vi "Skip Fire Write.vi"(0 "Device Inputs":dbl[](array[numeric]), 11 "Setup Indexes":T2[](array[typedef])) -> (6 "Setup":T1[](array[typedef]))   [LabVIEW 2016, in "DCM Engine.lvlib"]
uses:
  DCM Engine.lvlib
  Shared/Types/Skip Fire Setup Indexes.ctl
  Built/DCM Classes Packed/Pharlap/C/DCM-Classes.lvlibp/DCM/Skip Fire/RT/Skip Fire Setup.ctl
  Built/DCM Classes Packed/Pharlap/C/DCM-Classes.lvlibp/DCM/Skip Fire/RT/DCM - RT - Skip Fire.lvlib
  DCM Shared.lvlib
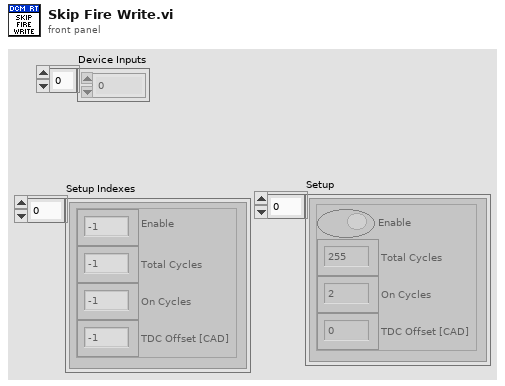
[diagram p1: front panel]
types:
  T1 = typedef "DCM-Classes.lvlibp/DCM - RT - Skip Fire.lvlib/Skip Fire Setup.ctl" = cluster{"Enable":bool, "Total Cycles":u8, "On Cycles":u8, "TDC Offset [CAD]":sgl}
  T2 = typedef "DCM Shared.lvlib/Skip Fire Setup Indexes.ctl" = cluster{"Enable":i32, "Total Cycles":i32, "On Cycles":i32, "TDC Offset [CAD]":i32}
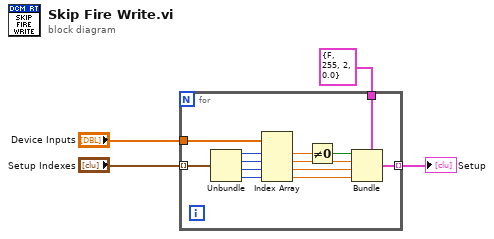
[diagram p0: block diagram]
diagram:
  n1 = for {
    tunnel: "Device Inputs" -> [w17]
    tunnel: "Setup Indexes" -> [w16] mode=indexing
    tunnel: T1 {"Enable"=FALSE, "Total Cycles"=255, "On Cycles"=2, "TDC Offset [CAD]"=0.0} ("Angle Control") -> [w11]
    tunnel: [w5] -> w1 mode=indexing
    n2 = Unbundle(w16) -> ("Enable"=w15:i32, "Total Cycles"=w14:i32, "On Cycles"=w13:i32, "TDC Offset [CAD]"=w12:i32)
    n3 = Index Array(array=w17, index #1=w15, index #2=w14, index #3=w13, index #4=w12) -> (element #1=w10:dbl, element #2=w8:dbl, element #3=w7:dbl, element #4=w6:dbl)
    n4 = Not Equal To 0?(x=w10) -> (x != 0?=w9:bool)
    n5 = Bundle(cluster=w11, "Enable"=w9, "Total Cycles"=w8, "On Cycles"=w7, "TDC Offset [CAD]"=w6) -> (w5:T1)
  }
  "Setup" <- w1
